vi "PH_Beckhoff-16BB_Testtool.set i attribute.vi"(0 "i ref in":refnum<vi>, 2 "i attribute":T1, 5 "error in (no error)":errorcluster) -> (14 "i ref out":refnum<vi>, 19 "error out":errorcluster)   [LabVIEW 2014, in "PH_Beckhoff-16BB_Testtool.lvlib"]
doc: "Sets the i attribute data of an object.\n\nLicense Agreement for this software:\n\nCopyright (C)\nGesellschaft für Schwerionenforschung, GSI\nPlanckstr. 1\n64291 Darmstadt\nGermany\n\nContact: D.Beck@gsi.de \n\nThis program is free software; you can redistribute it and/or modify it under the terms of the GNU General Public License as published by the Free Software Foundation; either version 2 of the license, or (at your option) any later version.\n\nThis program is distributed in the hope that it will be useful, but WITHOUT ANY WARRANTY; without even the implied warranty of MERCHANTABILITY or FITNESS FOR A PARTICULAR PURPOSE. See the GNU General License for more details (http://www.gnu.org).\n\nGesellschaft für Schwerionenforschung, GSI\nPlanckstr. 1, 64291 Darmstadt, Germany\nFor all questions and ideas contact: M.Richter@gsi.de, H.Brand@gsi.de or D.Beck@gsi.de.\nLast update: 17-JUN-2004"
uses:
  PH_Beckhoff-16BB_Testtool.lvlib
  PH_Beckhoff-16BB_Testtool.i attribute.ctl
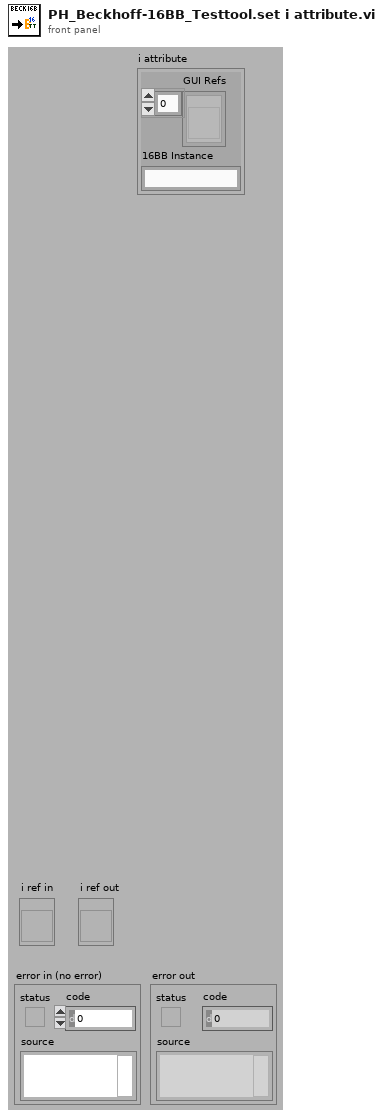
[diagram p1: front panel]
types:
  T1 = typedef "PH_Beckhoff-16BB_Testtool.lvlib/PH_Beckhoff-16BB_Testtool.i attribute.ctl" = cluster{"GUI Refs":refnum<vi>[], "16BB Instance":string}
  T2 = enum16{"SetAttribute", "GetAttribute", "CreateAttribute", "DestroyAttribute", "DestroyAllAtributes"}
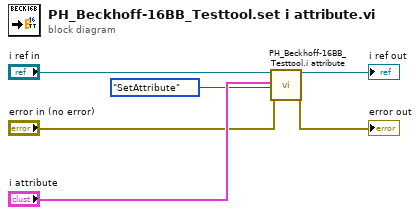
[diagram p0: block diagram]
diagram:
  n1 = call "PH_Beckhoff-16BB_Testtool.i attribute.vi"("VI Refnum"="i ref in", "CLASS.i attribute"="i attribute", "Action"=T2."SetAttribute", "error in (no error)"="error in (no error)") -> ("VI Refnum out"=→"i ref out":refnum<vi>, "error out"=→"error out":errorcluster)  [unwired: 13 in, 1 out]
